vi "SourceCoilControl_Wrapper.vi"(0 "Path Array":string[](array[string]), 1 "Input Values":dbl[](array[numeric])) -> ()   [LabVIEW 2018]
uses:
  <vilib>/Analysis/1siggen.llb/Ramp Pattern by Samples.vi
  <vilib>/DAQmx/write.llb/DAQmx Write (Analog 1D DBL 1Chan NSamp).vi
  <vilib>/DAQmx/create/channels.llb/DAQmx Create Channel (AO-Voltage-Basic).vi
  <vilib>/DAQmx/configure/timing.llb/DAQmx Timing (Sample Clock).vi
  <vilib>/DAQmx/miscellaneous.llb/DAQmx Fill In Error Info.vi
  <vilib>/Analysis/NI_AALBase.lvlib
panel:
  out "Time (s)":dbl
  out "Start Value":dbl
  out "EndValue":dbl
  out "Device name":string[](array[string])=["Dev1/ao1", "", "", "", ""]
  out "Set Values":dbl[](array[numeric])=[60.0, 7.5, 50.0, 0.0]
  out "Enable Source Coils?":bool
  in  "rate (S/s)":dbl=1000.0 format="%0.2f"
  in  "samples":i32=128
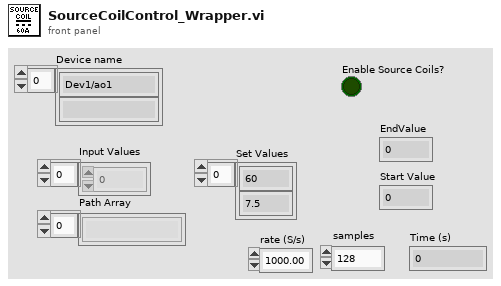
[diagram p1: front panel]
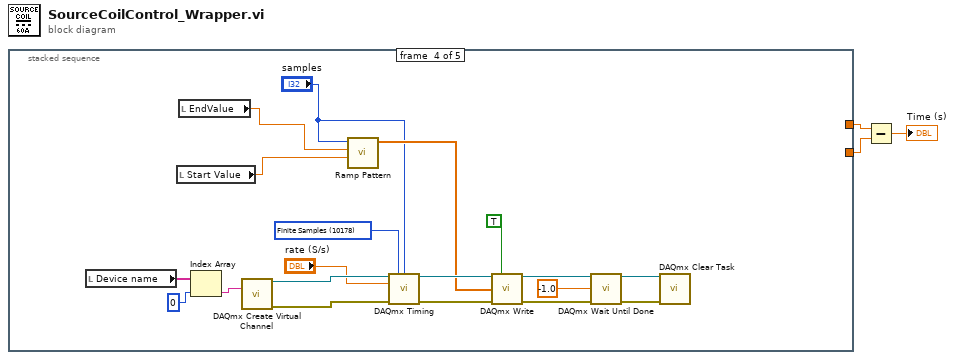
[diagram p0: block diagram]
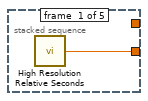
[diagram p2: hidden frame]
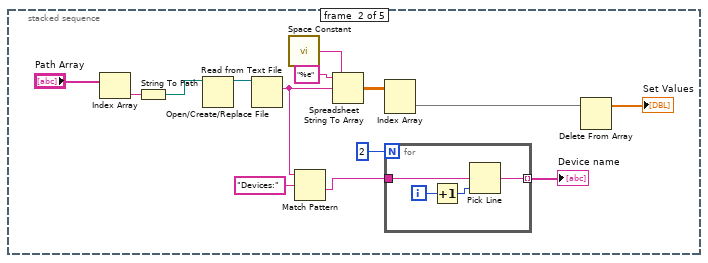
[diagram p3: hidden frame]
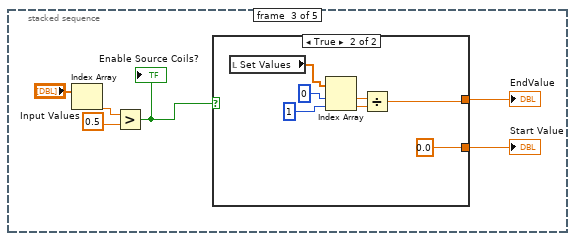
[diagram p4: hidden frame]
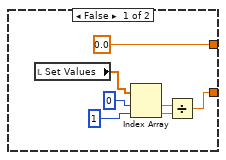
[diagram p5: hidden frame]
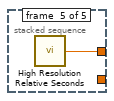
[diagram p6: hidden frame]
diagram:
  n1 = stacked-sequence {
    tunnel: [w4 _ _ _ _] -> w2
    tunnel: [_ _ _ _ w62] -> w3
    frame #0 {
      n2 = call <vilib>:"High Resolution Relative Seconds.vi"() -> ("relative seconds"=w4:dbl)
    }
    frame #1 {
      n3 = Index Array(array="Path Array") -> (element=w18:string)  [unwired: 1 in]
      n4 = String To Path(string=w18) -> (path=w6:path)
      n5 = Open/Create/Replace File(file path (use dialog)=w6) -> (refnum out=w8:refnum<file>)  [unwired: 5 in, 2 out]
      n6 = Read from Text File(file (use dialog)=w8) -> (text=w13:string)  [unwired: 3 in, 3 out]
      n7 = call <vilib>:"Space Constant.vi"() -> ("String"=w15:string)
      n8 = Match Pattern(string=w13, regular expression="Devices:") -> (after substring=w11:string)  [unwired: 1 in, 3 out]
      n9 = Spreadsheet String To Array(delimiter (Tab)=w15, format string="%e", spreadsheet string=w13) -> (array=w14:dbl[][])  [unwired: 1 in]
      n10 = Index Array(array=w14) -> (element=w9:dbl[])  [unwired: 2 in]
      n11 = for {
        N: 2 -> [_]
        tunnel: w11 -> [w20]
        tunnel: [w19] -> w5 mode=indexing
        i -> [w22]
        n12 = Increment(x=w22) -> (x+1=w21:i32)
        n13 = Pick Line(multi-line string=w20, line index=w21) -> (output string=w19:string)  [unwired: 1 in]
      }
      "Device name" <- w5
      n14 = Delete From Array(array=w9) -> (array with subset deleted=→"Set Values":dbl[])  [unwired: 2 in, 1 out]
    }
    frame #2 {
      n15 = Index Array(array="Input Values") -> (element=w27:dbl)  [unwired: 1 in]
      n16 = Greater?(x=w27, y=0.5) -> (0:w25:bool)
      "Enable Source Coils?" <- w25
      n17 = case shown="True" w25 {
        tunnel: [0.0 w37] -> w24
        tunnel: [w29 0.0] -> w23
        frame False {
          n18 = local read "Set Values"() -> (w34:dbl[])
          n19 = Index Array(array=w34, index #1=0 ("index"), index #2=1 ("index")) -> (element #1=w30:dbl, element #2=w31:dbl)
          n20 = Divide(x=w30, y=w31) -> (x/y=w29:dbl)
        }
        frame True {
          n21 = local read "Set Values"() -> (w42:dbl[])
          n22 = Index Array(array=w42, index #1=0 ("index"), index #2=1 ("index")) -> (element #1=w38:dbl, element #2=w39:dbl)
          n23 = Divide(x=w38, y=w39) -> (x/y=w37:dbl)
        }
      }
      "EndValue" <- w24
      "Start Value" <- w23
    }
    frame #3 {
      w49 = 10178 items=["Finite Samples"=10178, "Continuous Samples"=10123, "Hardware Timed Single Point"=12522] ("sample mode")
      n24 = local read "Device name"() -> (w45:string[])
      n25 = local read "Start Value"() -> (w46:dbl)
      n26 = local read "EndValue"() -> (w47:dbl)
      n27 = Index Array(array=w45, index=0) -> (element=w44:string)
      n28 = call-poly <vilib>:"DAQmx Create Virtual Channel.vi"("physical channels"=w44) -> ("task out"=w57:refnum<k21>, "error out"=w58:errorcluster)  [unwired: 13 in]
      n29 = call-poly <vilib>:"Ramp Pattern.vi"("start"=w46, "end"=w47, "samples"="samples") -> ("Ramp Pattern"=w50:dbl[])  [unwired: 7 in, 1 out]
      n30 = call-poly <vilib>:"DAQmx Timing.vi"("task/channels in"=w57, "sample mode"=w49, "samples per channel"="samples", "rate"="rate (S/s)", "error in"=w58) -> ("task out"=w60:refnum<k21>, "error out"=w59:errorcluster)  [unwired: 9 in]
      n31 = call-poly <vilib>:"DAQmx Write.vi"("task/channels in"=w60, "auto start"=TRUE, "data"=w50, "error in"=w59) -> ("task out"=w56:refnum<k21>, "error out"=w55:errorcluster)  [unwired: 9 in, 1 out]
      n32 = call <vilib>:"DAQmx Wait Until Done.vi"("task/channels in"=w56, "timeout (sec)"=-1.0, "error in"=w55) -> ("task out"=w54:refnum<k21>, "error out"=w53:errorcluster)  [unwired: 11 in]
      n33 = call <vilib>:"DAQmx Clear Task.vi"("task in"=w54, "error in"=w53) -> ()  [unwired: 13 in, 1 out]
    }
    frame #4 {
      n34 = call <vilib>:"High Resolution Relative Seconds.vi"() -> ("relative seconds"=w62:dbl)
    }
  }
  n35 = Subtract(x=w3, y=w2) -> (x-y=→"Time (s)":dbl)
